vi "SIP_day002.vi"() -> ()   [LabVIEW 2025]
panel:
  in  "B factor":dbl(slide) scale=0.0..1000.0
  in  "Enum":enum16{"Morlet Wavelet", "damp sine"}(ring)
  in  "stop":bool
  out "Waveform Graph 2":dbl[](graph)
  in  "NP 2":dbl(slide) scale=0.0..10.0
  in  "N 2":i32(slide) scale=0.0..1000.0
  in  "Amplitude A 2":dbl(slide) scale=0.0..10.0
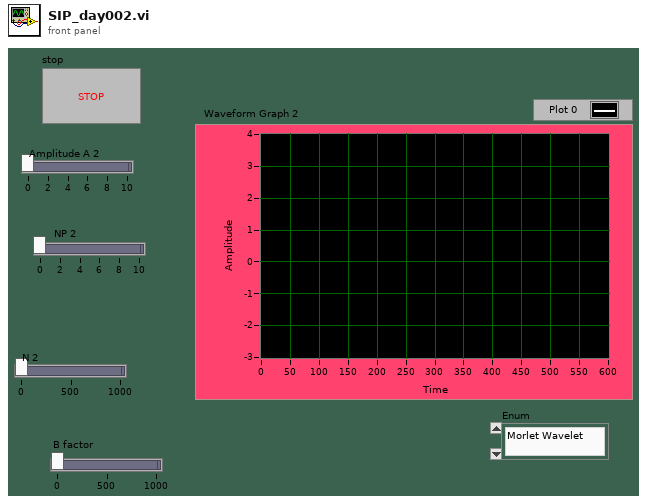
[diagram p1: front panel]
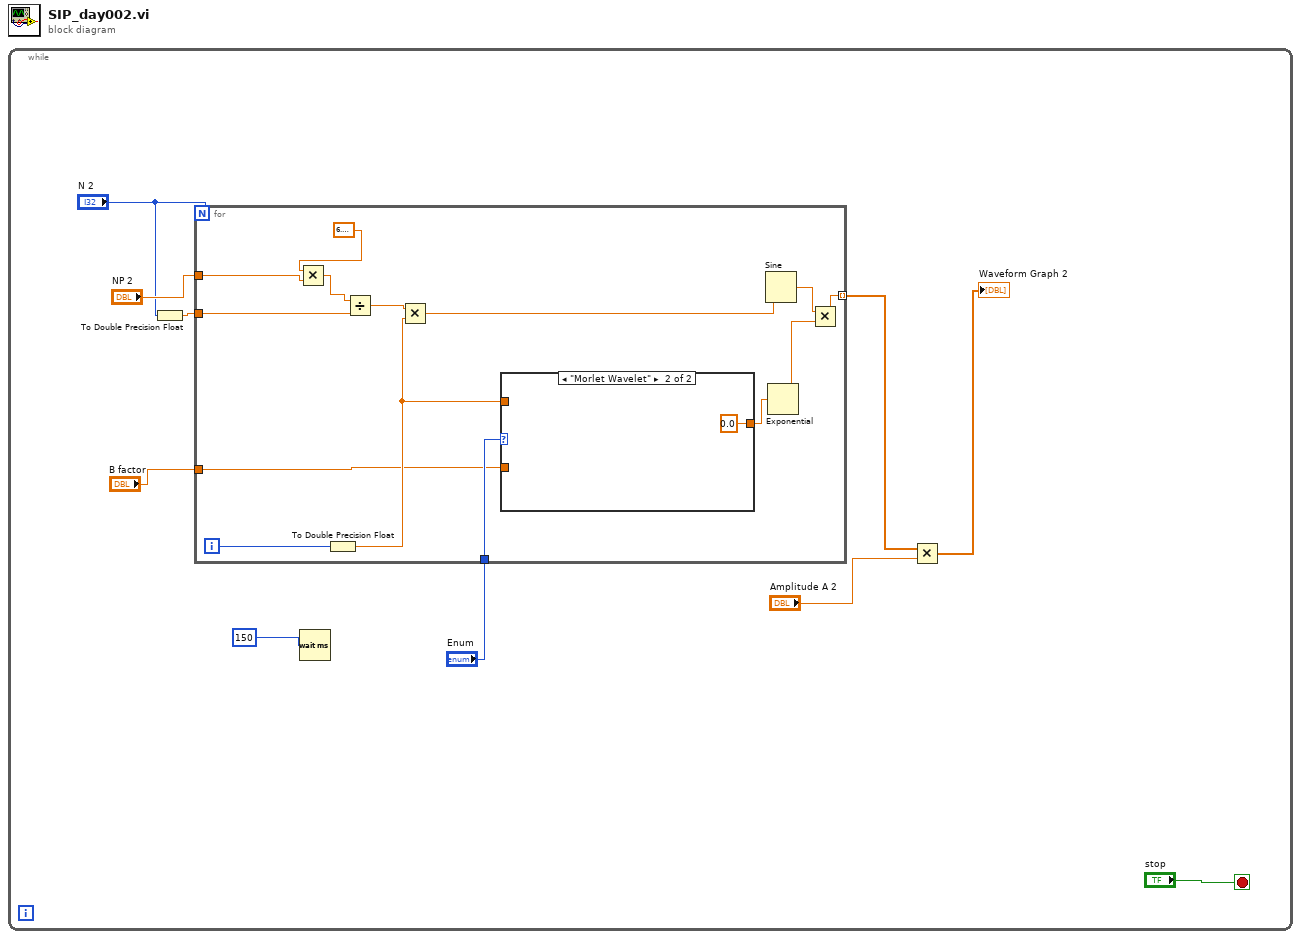
[diagram p0: block diagram]
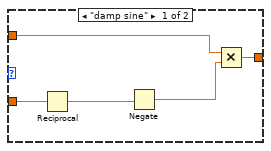
[diagram p2: hidden frame]
diagram:
  n1 = while {
    stop <- "stop" stop-if-true
    n2 = To Double Precision Float(number="N 2") -> (double precision float=w8:dbl)
    n3 = for {
      N: "N 2" -> [_]
      tunnel: "NP 2" -> [w24]
      tunnel: w8 -> [w22]
      tunnel: [w11] -> w6 mode=indexing
      tunnel: "Enum" -> [w17]
      tunnel: "B factor" -> [w15]
      i -> [w20]
      n4 = Multiply(x=6.283185307179586, y=w24) -> (x*y=w23:dbl)
      n5 = To Double Precision Float(number=w20) -> (double precision float=w16:dbl)
      n6 = Divide(x=w23, y=w22) -> (x/y=w21:dbl)
      n7 = Multiply(x=w21, y=w16) -> (x*y=w19:dbl)
      n8 = case shown="\"Morlet Wavelet\"" w17 {
        tunnel: w16 -> [w29 _]
        tunnel: w15 -> [w28 _]
        tunnel: [w25 0.0] -> w14
        frame "damp sine" {
          n9 = Reciprocal(x=w28) -> (1/x=w27:dbl)
          n10 = Negate(x=w27) -> (-x=w26:dbl)
          n11 = Multiply(x=w29, y=w26) -> (x*y=w25:dbl)
        }
        frame "Morlet Wavelet" {
        }
      }
      n12 = Sine(x=w19) -> (sin(x)=w13:dbl)
      n13 = Exponential(1:w14) -> (0:w12:dbl)
      n14 = Multiply(x=w13, y=w12) -> (x*y=w11:dbl)
    }
    n15 = Wait (ms)(milliseconds to wait=u32 150 ("millisecond timer value")) -> ()  [unwired: 1 out]
    n16 = Multiply(x=w6, y="Amplitude A 2") -> (x*y=→"Waveform Graph 2":dbl[])
  }
